vi "tcs testing sandbox.vi"   [LabVIEW 2022 SP3]
uses:
  TCS/TCS_external_interfaces/TCSDataDefinitions/TCSCommand/TargetConfiguration/Target/FixedTarget/RADecTarget/RADecTarget.lvclass
  TCS/TCS_external_interfaces/TCSDataDefinitions/TCSCommand/TargetConfiguration/Target/FixedTarget/RADecParameters/RADecParameters.lvclass
  TCS/TCS_external_interfaces/TCSDataDefinitions/TCSCommand/TargetConfiguration/Target/FixedTarget/Declination/Declination.lvclass
  TCS/TCS_external_interfaces/TCSDataDefinitions/TCSPublicStatus/CurrentTimes/ClockTimes/ClockTimes.lvclass
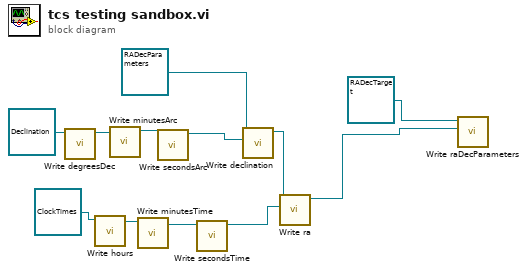
[diagram p0: block diagram]
diagram:
  n1 = call "Write degreesDec.vi"("Declination in"=refnum<class "Declination.lvclass"> refnum) -> ("Declination out"=w10:refnum<class "Declination.lvclass">)  [unwired: 9 in, 1 out]
  n2 = call "Write hours.vi"("ClockTimes in"=refnum<class "ClockTimes.lvclass"> refnum ("TCSDataDefinitions.lvlib:TCSPublicStatus.lvlib:CurrentTimes.lvlib:ClockTimes.lvclass")) -> ("ClockTimes out"=w6:refnum<class "ClockTimes.lvclass">)  [unwired: 9 in, 1 out]
  n3 = call "Write minutesArc.vi"("Declination in"=w10) -> ("Declination out"=w9:refnum<class "Declination.lvclass">)  [unwired: 9 in, 1 out]
  n4 = call "Write minutesTime.vi"("ClockTimes in"=w6) -> ("ClockTimes out"=w5:refnum<class "ClockTimes.lvclass">)  [unwired: 9 in, 1 out]
  n5 = call "Write secondsArc.vi"("Declination in"=w9) -> ("Declination out"=w8:refnum<class "Declination.lvclass">)  [unwired: 9 in, 1 out]
  n6 = call "Write secondsTime.vi"("ClockTimes in"=w5) -> ("ClockTimes out"=w4:refnum<class "ClockTimes.lvclass">)  [unwired: 9 in, 1 out]
  n7 = call "Write declination.vi"("Declination.lvclass"=w8, "RADecParameters in"=refnum<class "RADecParameters.lvclass"> refnum) -> ("RADecParameters out"=w2:refnum<class "RADecParameters.lvclass">)  [unwired: 8 in, 1 out]
  n8 = call "Write ra.vi"("ClockTimes.lvclass"=w4, "RADecParameters in"=w2) -> ("RADecParameters out"=w3:refnum<class "RADecParameters.lvclass">)  [unwired: 8 in, 1 out]
  n9 = call "Write raDecParameters.vi"("RADecParameters.lvclass"=w3, "RADecTarget in"=refnum<class "RADecTarget.lvclass"> refnum ("TCSDataDefinitions.lvlib:TCSCommand.lvlib:TargetConfiguration.lvlib:Target.lvlib:FixedTarget.lvlib:RADecTarget.lvclass")) -> ()  [unwired: 8 in, 2 out]
